vi "Initialize.vi"(6 "Actor Name":string, 7 "Host Name":string, 8 "error in (no error)":errorcluster, 11 "Message Broker Interface":refnum<class "Message Broker Interface.lvclass">) -> (0 "error out":errorcluster, 3 "Car Wash Display out":refnum<class "Car Wash Display.lvclass">)   [LabVIEW 2016, in "CLD Exam - Car Wash.lvlib" / "Car Wash Display.lvclass"]
uses:
  Car Wash Display.lvclass
  D:/Repos/Stream/software/Mediator/Classes/Mediated Actor/Mediated Actor.lvclass
  Mediator/Classes/Message Broker Interface/Message Broker Interface.lvclass
  Mediator/Classes/Message Interface/Message Interface.lvclass
  Mediator/Classes/Message Transport Queue/Message Transport Queue.lvclass
  Mediator/Classes/Mediated Actor/Mediated Actor.lvclass
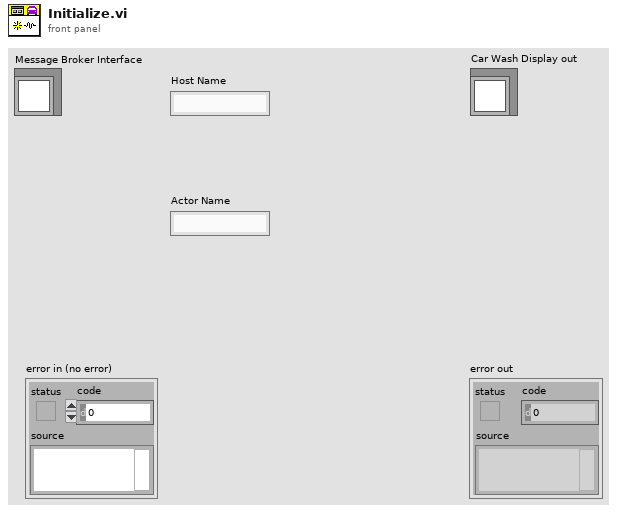
[diagram p1: front panel]
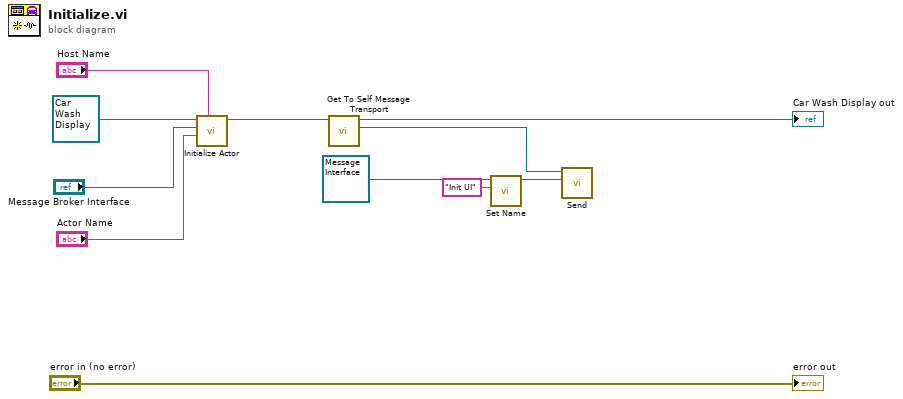
[diagram p0: block diagram]
diagram:
  n1 = call-dynamic "Initialize Actor.vi"("Host Name"="Host Name", "Actor Name"="Actor Name", "Message Broker Interface"="Message Broker Interface", "Car Wash Console in"=refnum<class "Car Wash Display.lvclass"> refnum ("Car Wash Display in")) -> ("Car Wash Console out"=w6:refnum<class "Car Wash Display.lvclass">)  [unwired: 6 in, 1 out]
  n2 = call "Get To Self Message Transport.vi"("Mediated Actor in"=w6) -> ("To Self"=w2:refnum<class "Message Transport Queue.lvclass">, "Mediated Actor out"=→"Car Wash Display out":refnum<class "Car Wash Display.lvclass">)  [unwired: 9 in]
  n3 = call "Set Name.vi"("Name"="Init UI", "Message Interface in"=refnum<class "Message Interface.lvclass"> refnum) -> ("Message Interface out"=w3:refnum<class "Message Interface.lvclass">)  [unwired: 8 in, 1 out]
  n4 = call-dynamic "Send.vi"("Message"=w3, "Message Transport Queue in"=w2) -> ()  [unwired: 7 in, 3 out]
  "error out" <- "error in (no error)"
